vi "Drums Only.vi"() -> ()   [LabVIEW 2009]
uses:
  <vilib>/vision/Image Controls.llb/IMAQ Image.ctl
  <vilib>/Instr/_visa.llb/VISA Configure Serial Port (Instr).vi
  <vilib>/Analysis/3filter.llb/Filter Passband Type.ctl
  <vilib>/Analysis/3filter.llb/Butterworth Filter (DBL).vi
  <vilib>/vision/NI_Vision_Development_Module.lvlib
  <vilib>/Analysis/NI_AALBase.lvlib
panel:
  in  "Orange Guitar":T1={"Global Rectangle"=[220, 296, 225, 371], "Contours"=[{"ID"=enum."External", "Type"=2, "Coordinates"=[224, 370, 220, 296]}]} {"Contours"."Type" items=["No Selection", "Point", "Line", "Rectangle", "Oval", "Polygon", "Freehand Region", "Annulus", "Unused2", "Unused3", "Broken Line", "Freehand Line", "Rotated Rectangle"]}
  out "Orange Guitar":dbl[](graph)
  out "Orange Guitar LED":bool
  in  "sampling 8":dbl=1.0 format="%0.2f"
  in  "high 9":dbl=60.0 format="%0.2f"
  in  "low  8":dbl=0.12500000000000006 format="%0.4f"
  out "Orange Guitar":T1={"Global Rectangle"=[300, 297, 320, 380], "Contours"=[{"ID"=enum."External", "Type"=2, "Coordinates"=[300, 379, 319, 297]}]} {"Contours"."Type" items=["No Selection", "Point", "Line", "Rectangle", "Oval", "Polygon", "Freehand Region", "Annulus", "Unused2", "Unused3", "Broken Line", "Freehand Line", "Rotated Rectangle"]}
  in  "Green Guitar":T1={"Global Rectangle"=[100, 292, 131, 371], "Contours"=[{"ID"=enum."External", "Type"=2, "Coordinates"=[100, 370, 130, 292]}]} {"Contours"."Type" items=["No Selection", "Point", "Line", "Rectangle", "Oval", "Polygon", "Freehand Region", "Annulus", "Unused2", "Unused3", "Broken Line", "Freehand Line", "Rotated Rectangle"]}
  in  "Blue Guitar":T1={"Global Rectangle"=[193, 293, 199, 374], "Contours"=[{"ID"=enum."External", "Type"=2, "Coordinates"=[193, 373, 198, 293]}]} {"Contours"."Type" items=["No Selection", "Point", "Line", "Rectangle", "Oval", "Polygon", "Freehand Region", "Annulus", "Unused2", "Unused3", "Broken Line", "Freehand Line", "Rotated Rectangle"]}
  in  "Red Guitar":T1={"Global Rectangle"=[129, 294, 154, 376], "Contours"=[{"ID"=enum."External", "Type"=2, "Coordinates"=[129, 375, 153, 294]}]} {"Contours"."Type" items=["No Selection", "Point", "Line", "Rectangle", "Oval", "Polygon", "Freehand Region", "Annulus", "Unused2", "Unused3", "Broken Line", "Freehand Line", "Rotated Rectangle"]}
  in  "Yellow Guitar":T1={"Global Rectangle"=[160, 295, 175, 378], "Contours"=[{"ID"=enum."External", "Type"=2, "Coordinates"=[160, 377, 174, 295]}]} {"Contours"."Type" items=["No Selection", "Point", "Line", "Rectangle", "Oval", "Polygon", "Freehand Region", "Annulus", "Unused2", "Unused3", "Broken Line", "Freehand Line", "Rotated Rectangle"]}
  in  "sampling  8":dbl=1.0 format="%0.2f"
  in  "high 8":dbl=60.0 format="%0.2f"
  out "Blue Guitar":dbl[](graph)
  in  "low 2":dbl=0.12500000000000006 format="%0.4f"
  out "Yellow Guitar":dbl[](graph)
  out "Yellow Guitar LED":bool
  in  "sampling 7":dbl=1.0 format="%0.2f"
  in  "high 7":dbl=60.0 format="%0.2f"
  in  "low  7":dbl=0.12500000000000006 format="%0.4f"
  out "Yellow Guitar":T1={"Global Rectangle"=[243, 262, 261, 384], "Contours"=[{"ID"=enum."External", "Type"=2, "Coordinates"=[260, 383, 243, 262]}]} {"Contours"."Type" items=["No Selection", "Point", "Line", "Rectangle", "Oval", "Polygon", "Freehand Region", "Annulus", "Unused2", "Unused3", "Broken Line", "Freehand Line", "Rotated Rectangle"]}
  out "Blue Guitar":T1={"Global Rectangle"=[168, 264, 180, 378], "Contours"=[{"ID"=enum."External", "Type"=2, "Coordinates"=[168, 377, 179, 264]}]} {"Contours"."Type" items=["No Selection", "Point", "Line", "Rectangle", "Oval", "Polygon", "Freehand Region", "Annulus", "Unused2", "Unused3", "Broken Line", "Freehand Line", "Rotated Rectangle"]}
  out "Green Guitar":dbl[](graph)
  out "Green Guitar LED":bool
  in  "sampling 6":dbl=1.0 format="%0.2f"
  in  "high 6":dbl=60.0 format="%0.2f"
  in  "low  6":dbl=0.12500000000000006 format="%0.4f"
  out "Green Guitar":T1={"Global Rectangle"=[406, 309, 423, 383], "Contours"=[{"ID"=enum."External", "Type"=2, "Coordinates"=[422, 382, 406, 309]}]} {"Contours"."Type" items=["No Selection", "Point", "Line", "Rectangle", "Oval", "Polygon", "Freehand Region", "Annulus", "Unused2", "Unused3", "Broken Line", "Freehand Line", "Rotated Rectangle"]}
  out "Red Guitar":dbl[](graph)
  out "Red Guitar LED":bool
  in  "sampling 5":dbl=1.0 format="%0.2f"
  in  "high 5":dbl=60.0 format="%0.2f"
  in  "low  5":dbl=0.12500000000000006 format="%0.4f"
  out "Red Guitar":T1={"Global Rectangle"=[300, 297, 320, 380], "Contours"=[{"ID"=enum."External", "Type"=2, "Coordinates"=[300, 379, 319, 297]}]} {"Contours"."Type" items=["No Selection", "Point", "Line", "Rectangle", "Oval", "Polygon", "Freehand Region", "Annulus", "Unused2", "Unused3", "Broken Line", "Freehand Line", "Rotated Rectangle"]}
  out "Blue Guitar LED":bool
  in  "Mask":T1 {"Contours"."Type" items=["No Selection", "Point", "Line", "Rectangle", "Oval", "Polygon", "Freehand Region", "Annulus", "Unused2", "Unused3", "Broken Line", "Freehand Line", "Rotated Rectangle"]}
  out "Image 2":T2(plugin-control)
  out "Red Line":T1={"Global Rectangle"=[300, 297, 320, 380], "Contours"=[{"ID"=enum."External", "Type"=2, "Coordinates"=[300, 379, 319, 297]}]} {"Contours"."Type" items=["No Selection", "Point", "Line", "Rectangle", "Oval", "Polygon", "Freehand Region", "Annulus", "Unused2", "Unused3", "Broken Line", "Freehand Line", "Rotated Rectangle"]}
  in  "Red Line":T1={"Global Rectangle"=[300, 297, 320, 380], "Contours"=[{"ID"=enum."External", "Type"=2, "Coordinates"=[300, 379, 319, 297]}]} {"Contours"."Type" items=["No Selection", "Point", "Line", "Rectangle", "Oval", "Polygon", "Freehand Region", "Annulus", "Unused2", "Unused3", "Broken Line", "Freehand Line", "Rotated Rectangle"]}
  out "Waveform Red":dbl[](graph)
  out "LED Red":bool
  in  "sampling 4":dbl=1.0 format="%0.2f"
  in  "high 4":dbl=60.0 format="%0.2f"
  in  "low  4":dbl=0.12500000000000006 format="%0.4f"
  out "Green Line":T1={"Global Rectangle"=[406, 309, 423, 383], "Contours"=[{"ID"=enum."External", "Type"=2, "Coordinates"=[422, 382, 406, 309]}]} {"Contours"."Type" items=["No Selection", "Point", "Line", "Rectangle", "Oval", "Polygon", "Freehand Region", "Annulus", "Unused2", "Unused3", "Broken Line", "Freehand Line", "Rotated Rectangle"]}
  in  "Blue Line":T1={"Global Rectangle"=[374, 278, 383, 377], "Contours"=[{"ID"=enum."External", "Type"=2, "Coordinates"=[382, 376, 374, 278]}]} {"Contours"."Type" items=["No Selection", "Point", "Line", "Rectangle", "Oval", "Polygon", "Freehand Region", "Annulus", "Unused2", "Unused3", "Broken Line", "Freehand Line", "Rotated Rectangle"]}
  in  "Green Line":T1={"Global Rectangle"=[406, 309, 423, 383], "Contours"=[{"ID"=enum."External", "Type"=2, "Coordinates"=[422, 382, 406, 309]}]} {"Contours"."Type" items=["No Selection", "Point", "Line", "Rectangle", "Oval", "Polygon", "Freehand Region", "Annulus", "Unused2", "Unused3", "Broken Line", "Freehand Line", "Rotated Rectangle"]}
  in  "low  3":dbl=0.12500000000000006 format="%0.4f"
  out "Waveform Green":dbl[](graph)
  out "LED Green":bool
  in  "sampling 3":dbl=1.0 format="%0.2f"
  in  "high 3":dbl=60.0 format="%0.2f"
  in  "Yellow Line":T1={"Global Rectangle"=[342, 292, 349, 377], "Contours"=[{"ID"=enum."External", "Type"=2, "Coordinates"=[342, 376, 348, 292]}]} {"Contours"."Type" items=["No Selection", "Point", "Line", "Rectangle", "Oval", "Polygon", "Freehand Region", "Annulus", "Unused2", "Unused3", "Broken Line", "Freehand Line", "Rotated Rectangle"]}
  out "Blue Line":T1={"Global Rectangle"=[168, 264, 180, 378], "Contours"=[{"ID"=enum."External", "Type"=2, "Coordinates"=[168, 377, 179, 264]}]} {"Contours"."Type" items=["No Selection", "Point", "Line", "Rectangle", "Oval", "Polygon", "Freehand Region", "Annulus", "Unused2", "Unused3", "Broken Line", "Freehand Line", "Rotated Rectangle"]}
  out "cluster":T3
  in  "baud rate (9600)":u32=9600
  in  "VISA resource name":refnum<visa-resource-name>
  out "number":u8
  out "decimal integer string":string
  out "Image Dst Out":T2
  out "Yellow Line":T1={"Global Rectangle"=[243, 262, 261, 384], "Contours"=[{"ID"=enum."External", "Type"=2, "Coordinates"=[260, 383, 243, 262]}]} {"Contours"."Type" items=["No Selection", "Point", "Line", "Rectangle", "Oval", "Polygon", "Freehand Region", "Annulus", "Unused2", "Unused3", "Broken Line", "Freehand Line", "Rotated Rectangle"]}
  in  "low  2":dbl=0.12500000000000006 format="%0.4f"
  in  "high 2":dbl=60.0 format="%0.2f"
  in  "sampling 2":dbl=1.0 format="%0.2f"
  out "LED Yellow":bool
  out "Waveform Yellow":dbl[](graph)
  in  "playtime":dbl=30.0
  out "Frame Number":i32
  in  "Frame Start":i32=2400
  out "Blue Drum":bool
  in  "low":dbl=0.12500000000000006 format="%0.4f"
  out "Blue Drum":dbl[](graph)
  in  "high":dbl=60.0 format="%0.2f"
  in  "sampling":dbl=1.0 format="%0.2f"
  in  "stop":bool
  in  "AVI Path":path
  # "BLUE"
  # "YELLOW"
  # "GREEN"
  # "RED"
  # "Drums"
  # "Guitar"
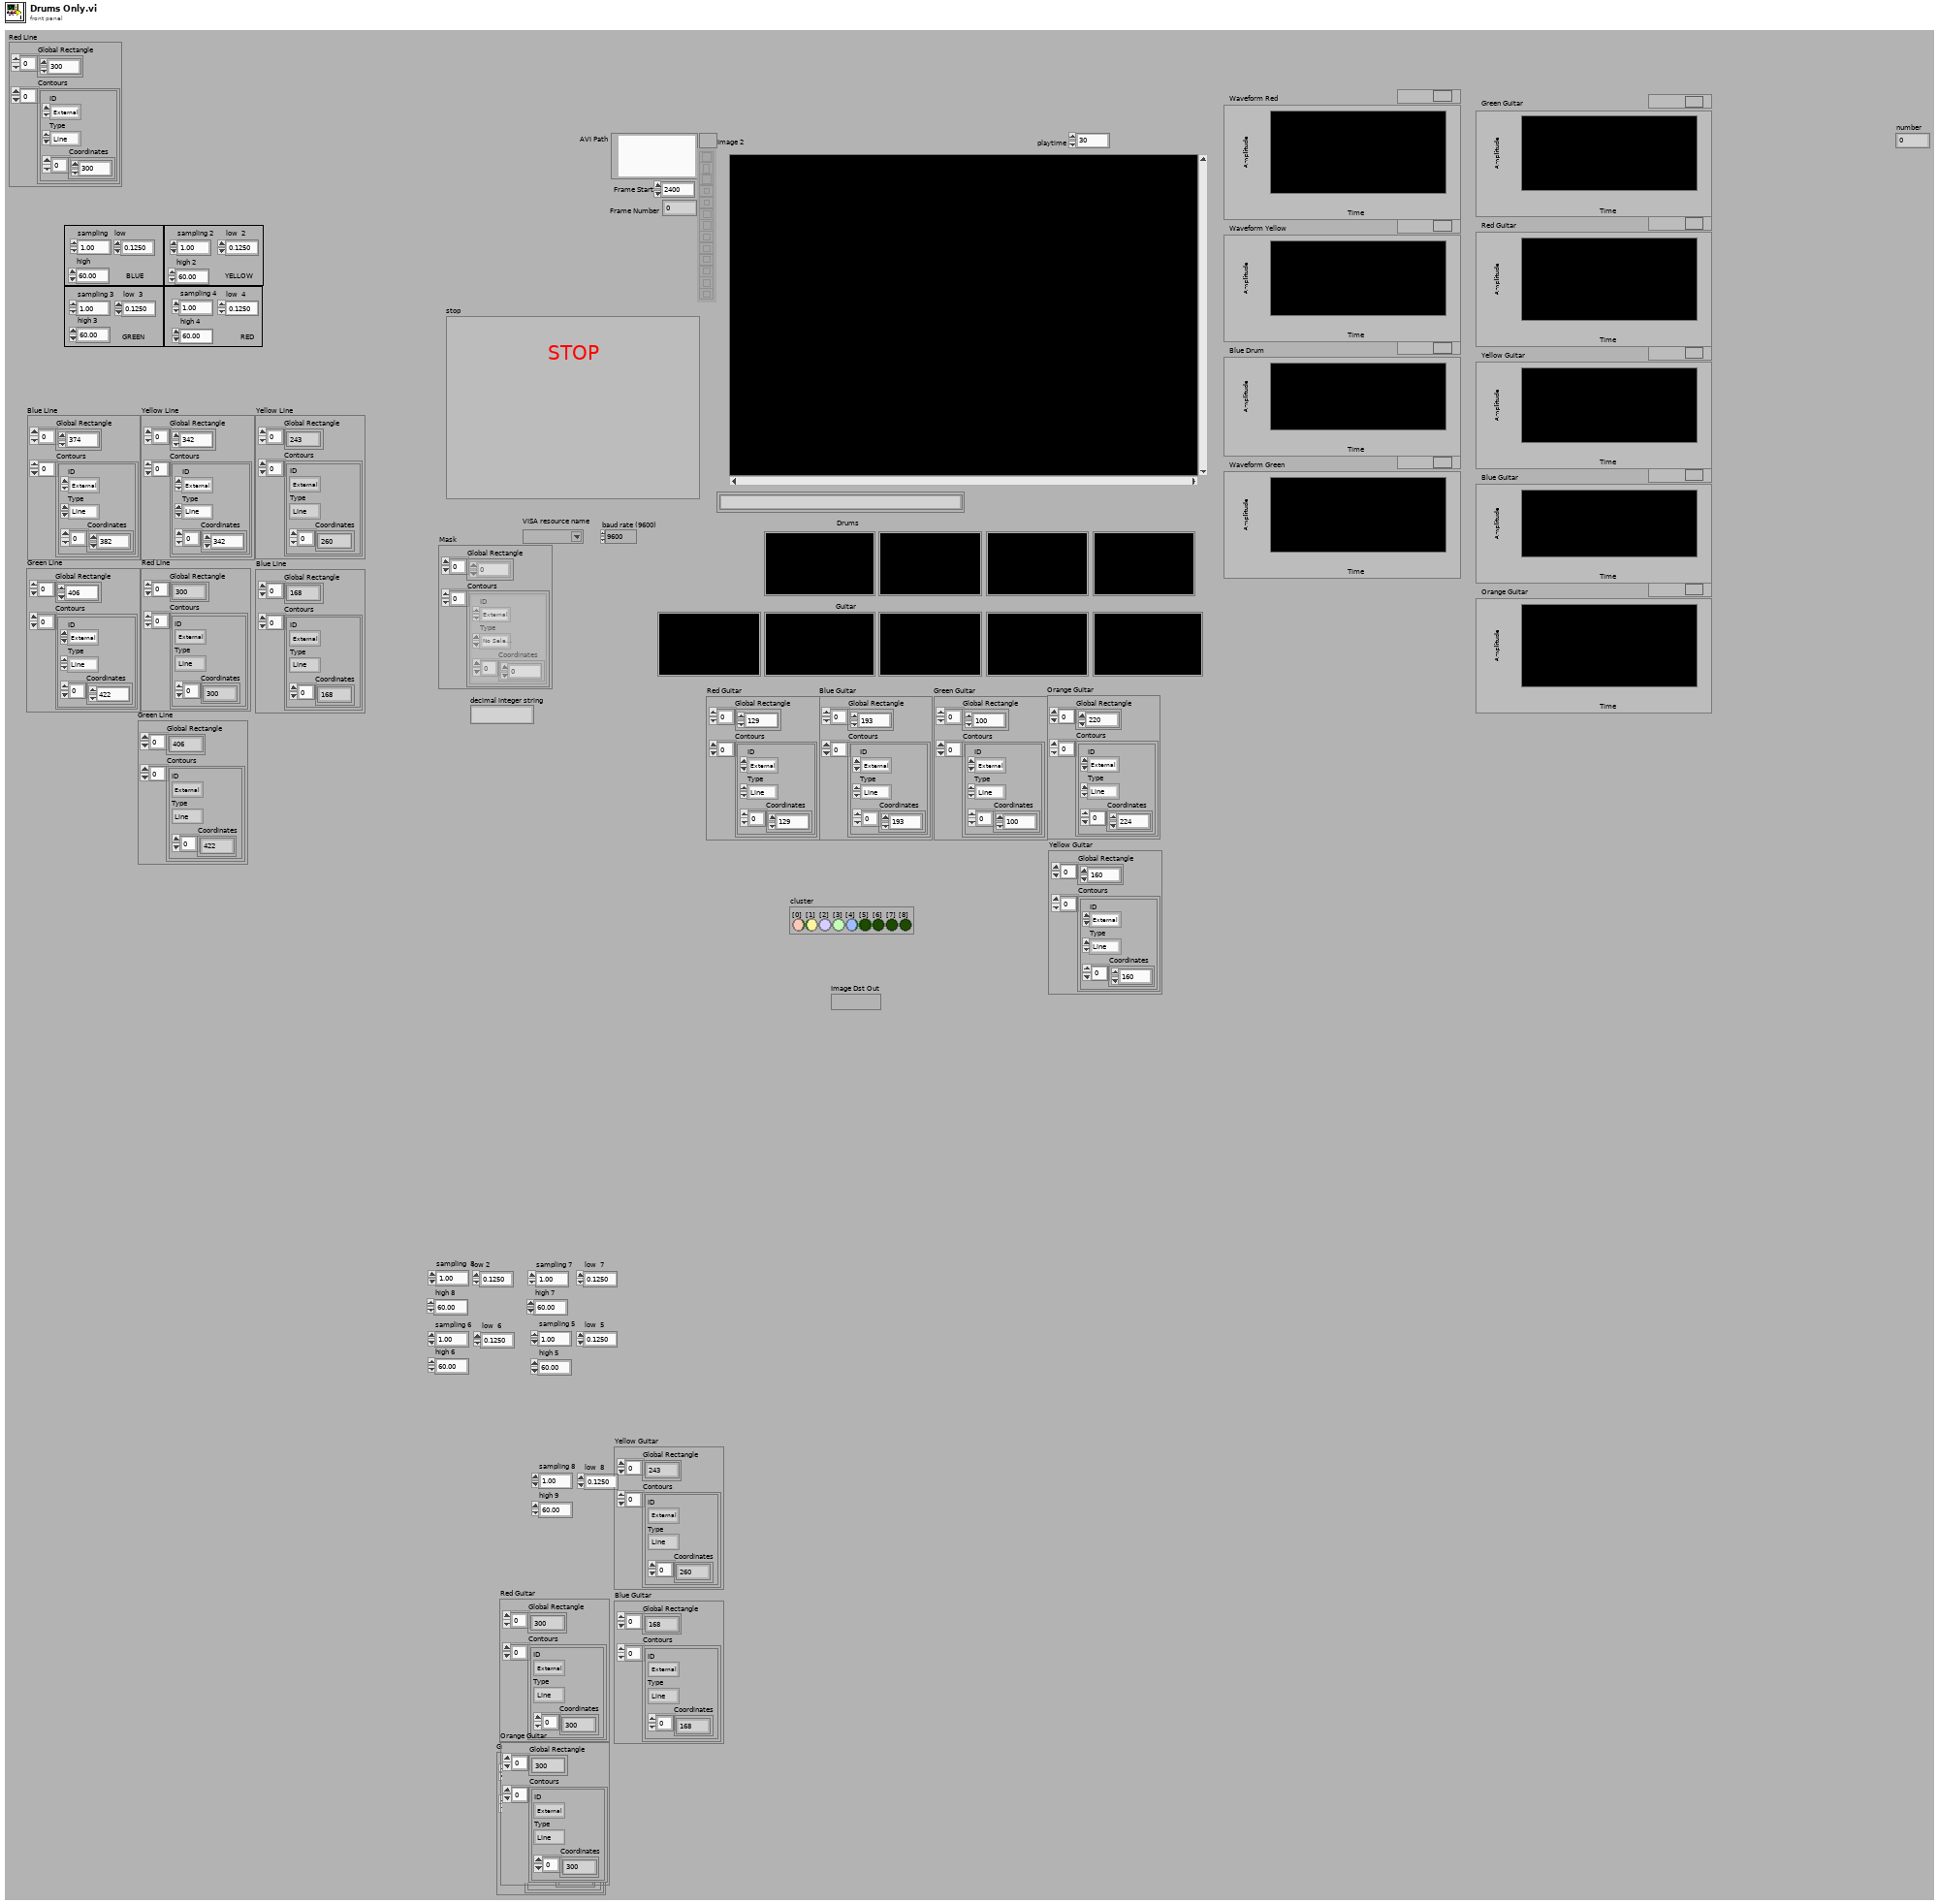
[diagram p1: front panel]
types:
  T1 = cluster{"Global Rectangle":i32[], "Contours":cluster{"ID":enum32{"External", "Internal"}, "Type":u32, "Coordinates":i32[]}[]}
  T2 = typedef "IMAQ Image.ctl" = refnum<image>
  T3 = cluster{"[0]":bool, "[1]":bool, "[2]":bool, "[3]":bool, "[4]":bool, "[5]":bool, "[6]":bool, "[7]":bool, "[8]":bool}
  T4 = typedef "NI_AALBase.lvlib/Filter Passband Type.ctl" = enum32{"Lowpass", "Highpass", "Bandpass", "Bandstop"}
  T5 = cluster{"Left":i32, "Top":i32, "Right":i32, "Bottom":i32}
  T6 = typedef "Image Type" = u32
  T7 = typedef "AviRefnum.ctl" = refnum<k1>
  T8 = cluster{"ID":enum32{"External", "Internal"}, "Type":u32, "Coordinates":i32[]}[]
  T9 = cluster{"ID":enum32{"External", "Internal"}, "Type":u32, "Coordinates":i32[]}
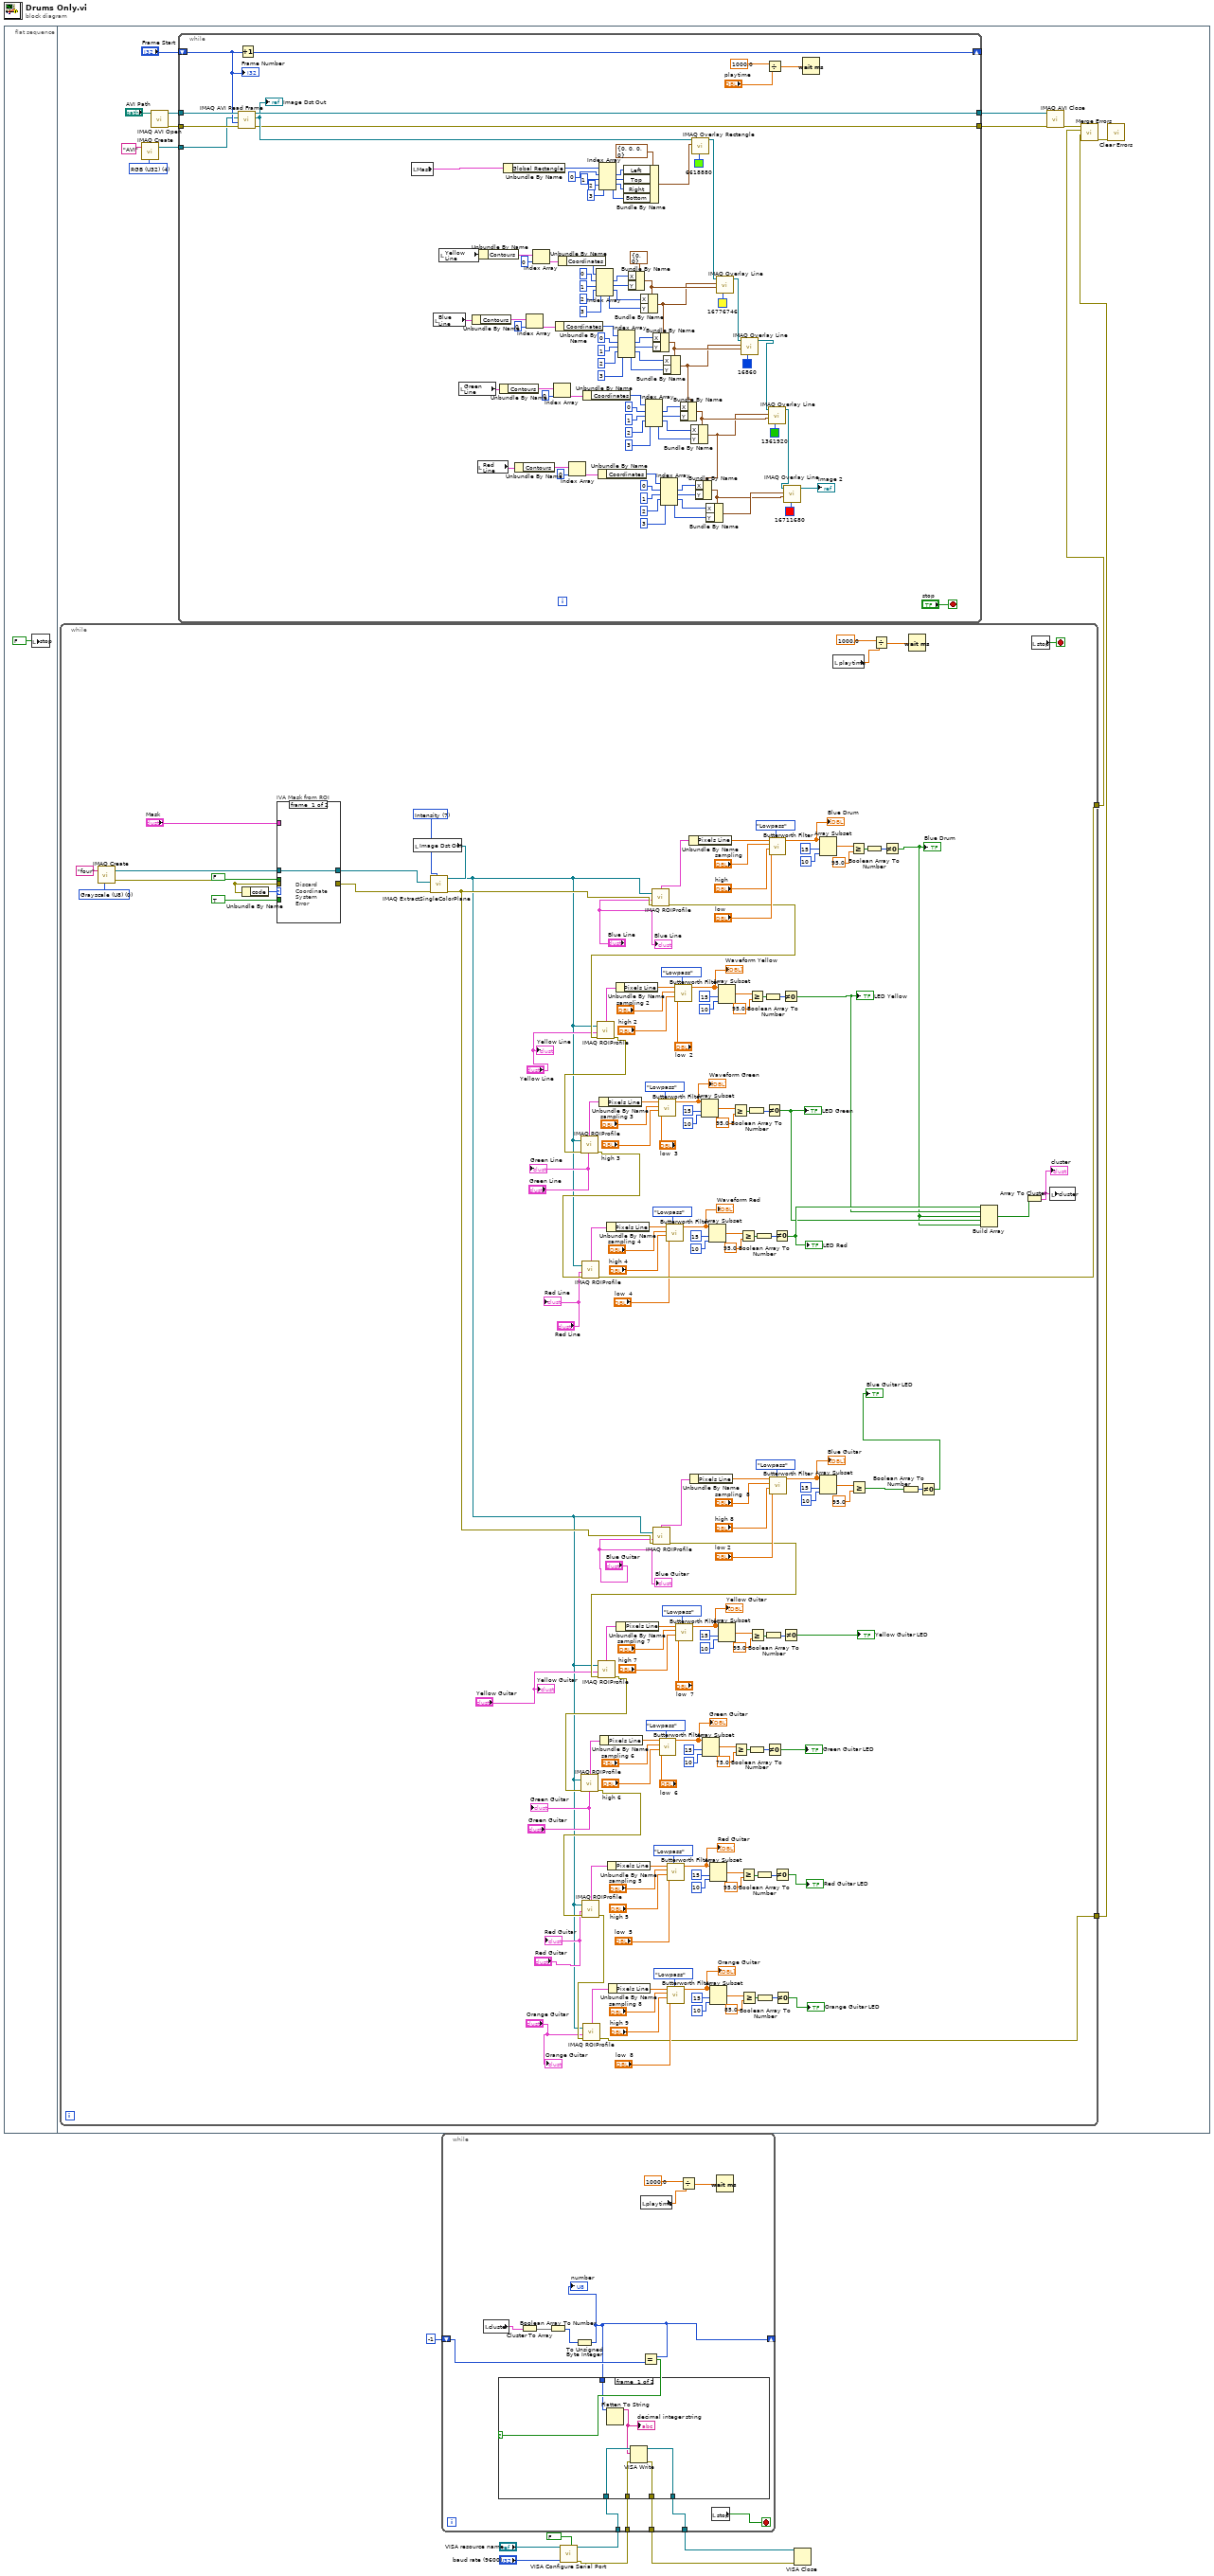
[diagram p0: block diagram]
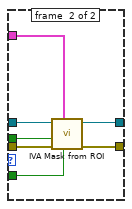
[diagram p3: hidden frame]
diagram:
  n1 = flat-sequence {
    frame #0 {
      n2 = local write "stop"(FALSE ("stop")) -> ()
    }
    frame #1 {
      w14 = T6 4 items=["Grayscale (U8)", "Grayscale (I16)", "Grayscale (SGL)", "Complex (CSG)", "RGB (U32)", "HSL (U32)", "RGB (U64)", "Grayscale (U16)"] ("Image Type")
      n3 = while {
        tunnel: [w170] -> w11
        tunnel: [w35] -> w10
        stop <- w185 stop-if-true
        w180 = T6 0 items=["Grayscale (U8)", "Grayscale (I16)", "Grayscale (SGL)", "Complex (CSG)", "RGB (U32)", "HSL (U32)", "RGB (U64)", "Grayscale (U16)"] ("Image Type")
        w186 = 7 items=["Red", "Green", "Blue", "Hue", "Saturation", "Luminance", "Value", "Intensity"] ("Color Plane")
        n4 = call "IMAQ Create"("Image Name"="four", "Image Type"=w180) -> ("New Image"=w173:T2, "error out"=w174:errorcluster)  [unwired: 3 in]
        n5 = Unbundle By Name(w174) -> ("code"=w178:i32)
        n6 = case "IVA Mask from ROI" shown="Default" w178 {
          tunnel: "Mask" -> [_ w194]
          tunnel: TRUE ("Shrink") -> [_ w193]
          tunnel: w173 -> [w187 w192]
          tunnel: w174 -> [_ w191]
          tunnel: [_ w190] -> w175
          tunnel: [w187 w189] -> w171
          tunnel: FALSE ("Out / In") -> [_ w188]
          frame #0 {
            # "Discard\nCoordinate\nSystem\nError"
          }
          frame #1 {
            n7 = call <vilib>:"IVA Mask from ROI.vi"("Shrink"=w193, "ROI Descriptor"=w194, "error in (no error)"=w191, "Out / In"=w188, "Image Src"=w192) -> ("error out"=w190:errorcluster, "Image Out"=w189:T2)  [unwired: 5 out]
          }
        }
        n8 = local read "Image Dst Out"() -> (w181:T2)
        n9 = call "IMAQ ExtractSingleColorPlane"("Color Plane"=w186, "error in (no error)"=w175, "Image Dst"=w171, "Image Src"=w181) -> ("error out"=w169:errorcluster, "Image Dst Out"=w34:T2)  [unwired: 6 out]
        n10 = call "IMAQ ROIProfile"("error in (no error)"=w169, "ROI Descriptor"="Blue Line", "Image"=w34) -> ("error out"=w144:errorcluster, "ROI Graph"=w143:cluster{"x0":sgl, "dx":sgl, "Pixels Line":sgl[]})  [unwired: 4 out]
        n11 = call "IMAQ ROIProfile"("error in (no error)"=w144, "ROI Descriptor"="Yellow Line", "Image"=w34) -> ("error out"=w111:errorcluster, "ROI Graph"=w147:cluster{"x0":sgl, "dx":sgl, "Pixels Line":sgl[]})  [unwired: 4 out]
        n12 = call "IMAQ ROIProfile"("error in (no error)"=w111, "ROI Descriptor"="Green Line", "Image"=w34) -> ("error out"=w114:errorcluster, "ROI Graph"=w141:cluster{"x0":sgl, "dx":sgl, "Pixels Line":sgl[]})  [unwired: 4 out]
        n13 = call "IMAQ ROIProfile"("error in (no error)"=w114, "ROI Descriptor"="Red Line", "Image"=w34) -> ("error out"=w170:errorcluster, "ROI Graph"=w116:cluster{"x0":sgl, "dx":sgl, "Pixels Line":sgl[]})  [unwired: 4 out]
        n14 = Unbundle By Name(w141) -> ("Pixels Line"=w138:sgl[])
        n15 = Unbundle By Name(w116) -> ("Pixels Line"=w119:sgl[])
        n16 = Unbundle By Name(w147) -> ("Pixels Line"=w150:sgl[])
        n17 = call "IMAQ ROIProfile"("error in (no error)"=w169, "ROI Descriptor"="Blue Guitar", "Image"=w34) -> ("error out"=w84:errorcluster, "ROI Graph"=w83:cluster{"x0":sgl, "dx":sgl, "Pixels Line":sgl[]})  [unwired: 4 out]
        n18 = call "IMAQ ROIProfile"("error in (no error)"=w84, "ROI Descriptor"="Yellow Guitar", "Image"=w34) -> ("error out"=w54:errorcluster, "ROI Graph"=w87:cluster{"x0":sgl, "dx":sgl, "Pixels Line":sgl[]})  [unwired: 4 out]
        n19 = call "IMAQ ROIProfile"("error in (no error)"=w54, "ROI Descriptor"="Green Guitar", "Image"=w34) -> ("error out"=w55:errorcluster, "ROI Graph"=w81:cluster{"x0":sgl, "dx":sgl, "Pixels Line":sgl[]})  [unwired: 4 out]
        n20 = call "IMAQ ROIProfile"("error in (no error)"=w55, "ROI Descriptor"="Red Guitar", "Image"=w34) -> ("error out"=w36:errorcluster, "ROI Graph"=w57:cluster{"x0":sgl, "dx":sgl, "Pixels Line":sgl[]})  [unwired: 4 out]
        n21 = call "IMAQ ROIProfile"("error in (no error)"=w36, "ROI Descriptor"="Orange Guitar", "Image"=w34) -> ("error out"=w35:errorcluster, "ROI Graph"=w48:cluster{"x0":sgl, "dx":sgl, "Pixels Line":sgl[]})  [unwired: 4 out]
        n22 = Unbundle By Name(w81) -> ("Pixels Line"=w78:sgl[])
        n23 = Unbundle By Name(w57) -> ("Pixels Line"=w60:sgl[])
        n24 = Unbundle By Name(w48) -> ("Pixels Line"=w45:sgl[])
        n25 = Unbundle By Name(w87) -> ("Pixels Line"=w90:sgl[])
        n26 = call-poly <vilib>:"Butterworth Filter.vi"("filter type"=Filter_Passband_Type."Lowpass", "low cutoff freq: fl"="low  3", "high cutoff freq: fh"="high 3", "sampling freq: fs"="sampling 3", "X"=w138) -> ("Filtered X"=w142:dbl[])  [unwired: 3 in, 1 out]
        "Waveform Green" <- w142
        n27 = call-poly <vilib>:"Butterworth Filter.vi"("filter type"=Filter_Passband_Type."Lowpass", "low cutoff freq: fl"="low  6", "high cutoff freq: fh"="high 6", "sampling freq: fs"="sampling 6", "X"=w78) -> ("Filtered X"=w82:dbl[])  [unwired: 3 in, 1 out]
        "Green Guitar" <- w82
        n28 = call-poly <vilib>:"Butterworth Filter.vi"("filter type"=Filter_Passband_Type."Lowpass", "low cutoff freq: fl"="low  4", "high cutoff freq: fh"="high 4", "sampling freq: fs"="sampling 4", "X"=w119) -> ("Filtered X"=w115:dbl[])  [unwired: 3 in, 1 out]
        "Waveform Red" <- w115
        n29 = call-poly <vilib>:"Butterworth Filter.vi"("filter type"=Filter_Passband_Type."Lowpass", "low cutoff freq: fl"="low  5", "high cutoff freq: fh"="high 5", "sampling freq: fs"="sampling 5", "X"=w60) -> ("Filtered X"=w56:dbl[])  [unwired: 3 in, 1 out]
        "Red Guitar" <- w56
        n30 = call-poly <vilib>:"Butterworth Filter.vi"("filter type"=Filter_Passband_Type."Lowpass", "low cutoff freq: fl"="low  8", "high cutoff freq: fh"="high 9", "sampling freq: fs"="sampling 8", "X"=w45) -> ("Filtered X"=w49:dbl[])  [unwired: 3 in, 1 out]
        "Orange Guitar" <- w49
        n31 = call-poly <vilib>:"Butterworth Filter.vi"("filter type"=Filter_Passband_Type."Lowpass", "low cutoff freq: fl"="low  2", "high cutoff freq: fh"="high 2", "sampling freq: fs"="sampling 2", "X"=w150) -> ("Filtered X"=w146:dbl[])  [unwired: 3 in, 1 out]
        "Waveform Yellow" <- w146
        n32 = call-poly <vilib>:"Butterworth Filter.vi"("filter type"=Filter_Passband_Type."Lowpass", "low cutoff freq: fl"="low  7", "high cutoff freq: fh"="high 7", "sampling freq: fs"="sampling 7", "X"=w90) -> ("Filtered X"=w86:dbl[])  [unwired: 3 in, 1 out]
        "Yellow Guitar" <- w86
        n33 = Unbundle By Name(w143) -> ("Pixels Line"=w167:sgl[])
        n34 = Unbundle By Name(w83) -> ("Pixels Line"=w106:sgl[])
        n35 = Array Subset(array=w142, index=15, length=10) -> (w133:dbl[])
        n36 = Array Subset(array=w82, index=15, length=10) -> (w73:dbl[])
        n37 = Array Subset(array=w115, index=15, length=10) -> (w124:dbl[])
        n38 = Array Subset(array=w56, index=15, length=10) -> (w65:dbl[])
        n39 = Array Subset(array=w49, index=15, length=10) -> (w40:dbl[])
        n40 = Array Subset(array=w146, index=15, length=10) -> (w155:dbl[])
        n41 = Array Subset(array=w86, index=15, length=10) -> (w95:dbl[])
        n42 = Greater Or Equal?(x=w133, y=95.0) -> (x >= y?=w135:bool[])
        n43 = Greater Or Equal?(x=w73, y=75.0) -> (x >= y?=w75:bool[])
        n44 = Greater Or Equal?(x=w124, y=95.0) -> (x >= y?=w122:bool[])
        n45 = Greater Or Equal?(x=w65, y=95.0) -> (x >= y?=w63:bool[])
        n46 = Greater Or Equal?(x=w40, y=85.0) -> (x >= y?=w42:bool[])
        n47 = Boolean Array To Number(Boolean array=w135) -> (number=w136:u32)
        n48 = Greater Or Equal?(x=w155, y=95.0) -> (x >= y?=w153:bool[])
        n49 = Boolean Array To Number(Boolean array=w75) -> (number=w76:u32)
        n50 = Greater Or Equal?(x=w95, y=95.0) -> (x >= y?=w93:bool[])
        n51 = Boolean Array To Number(Boolean array=w122) -> (number=w121:u32)
        n52 = Boolean Array To Number(Boolean array=w63) -> (number=w62:u32)
        n53 = Boolean Array To Number(Boolean array=w42) -> (number=w43:u32)
        n54 = Boolean Array To Number(Boolean array=w153) -> (number=w152:u32)
        n55 = Boolean Array To Number(Boolean array=w93) -> (number=w92:u32)
        n56 = Not Equal To 0?(x=w136) -> (x != 0?=w24:bool)
        "LED Green" <- w24
        n57 = Not Equal To 0?(x=w76) -> (x != 0?=→"Green Guitar LED":bool)
        n58 = call-poly <vilib>:"Butterworth Filter.vi"("filter type"=Filter_Passband_Type."Lowpass", "low cutoff freq: fl"="low", "high cutoff freq: fh"="high", "sampling freq: fs"="sampling", "X"=w167) -> ("Filtered X"=w129:dbl[])  [unwired: 3 in, 1 out]
        "Blue Drum" <- w129
        n59 = call-poly <vilib>:"Butterworth Filter.vi"("filter type"=Filter_Passband_Type."Lowpass", "low cutoff freq: fl"="low 2", "high cutoff freq: fh"="high 8", "sampling freq: fs"="sampling  8", "X"=w106) -> ("Filtered X"=w69:dbl[])  [unwired: 3 in, 1 out]
        "Blue Guitar" <- w69
        n60 = Not Equal To 0?(x=w121) -> (x != 0?=w26:bool)
        "LED Red" <- w26
        n61 = Not Equal To 0?(x=w62) -> (x != 0?=→"Red Guitar LED":bool)
        n62 = Not Equal To 0?(x=w43) -> (x != 0?=→"Orange Guitar LED":bool)
        n63 = Not Equal To 0?(x=w152) -> (x != 0?=w25:bool)
        "LED Yellow" <- w25
        n64 = Not Equal To 0?(x=w92) -> (x != 0?=→"Yellow Guitar LED":bool)
        n65 = Array Subset(array=w129, index=15, length=10) -> (w161:dbl[])
        n66 = Array Subset(array=w69, index=15, length=10) -> (w100:dbl[])
        n67 = local read "playtime"() -> (w182:dbl)
        n68 = Greater Or Equal?(x=w161, y=95.0) -> (x >= y?=w159:bool[])
        n69 = Greater Or Equal?(x=w100, y=95.0) -> (x >= y?=w27:bool[])
        n70 = Boolean Array To Number(Boolean array=w159) -> (number=w158:u32)
        n71 = Divide(x=1000.0, y=w182) -> (x/y=w184:dbl)
        n72 = Not Equal To 0?(x=w158) -> (x != 0?=w23:bool)
        "Blue Drum" <- w23
        n73 = Boolean Array To Number(Boolean array=w27) -> (number=w98:u32)
        n74 = Wait (ms)(milliseconds to wait=w184) -> ()  [unwired: 1 out]
        n75 = Not Equal To 0?(x=w98) -> (x != 0?=→"Blue Guitar LED":bool)
        n76 = Build Array(w26, w25, w23, w24, w23) -> (w109:bool[])
        n77 = Array To Cluster(array=w109) -> (cluster=w110:T3)
        "cluster" <- w110
        n78 = local read "stop"() -> (w185:bool)
        n79 = local write "cluster"(w110) -> ()
        "Yellow Line" <- "Yellow Line"
        "Blue Line" <- "Blue Line"
        "Green Line" <- "Green Line"
        "Red Line" <- "Red Line"
        "Yellow Guitar" <- "Yellow Guitar"
        "Blue Guitar" <- "Blue Guitar"
        "Green Guitar" <- "Green Guitar"
        "Red Guitar" <- "Red Guitar"
        "Orange Guitar" <- "Orange Guitar"
      }
      n80 = call "IMAQ Create"("Image Name"="AVI", "Image Type"=w14) -> ("New Image"=w12:T2)  [unwired: 3 in, 1 out]
      n81 = call "IMAQ AVI Open"("AVI Path"="AVI Path") -> ("error out"=w19:errorcluster, "Avi Refnum"=w20:T7)  [unwired: 9 in]
      n82 = while {
        tunnel: w20 -> [w289]
        tunnel: w19 -> [w237]
        tunnel: [w288] -> w21
        shift-right: [w283] -> _
        shift-left: "Frame Start" -> [w282]
        tunnel: [w233] -> w15
        tunnel: w12 -> [w232]
        stop <- "stop" stop-if-true
        n83 = call "IMAQ AVI Read Frame"("error in (no error)"=w237, "Frame Number"=w282, "Image"=w232, "Avi Refnum"=w289) -> ("error out"=w233:errorcluster, "Image Out"=w234:T2, "Avi Refnum (duplicate)"=w288:T7)  [unwired: 4 in, 1 out]
        "Image Dst Out" <- w234
        n84 = Increment(x=w282) -> (x+1=w283:i32)
        n85 = local read "Mask"() -> (w195:T1)
        n86 = local read "Blue Line"() -> (w236:T1)
        n87 = local read "Yellow Line"() -> (w235:T1)
        n88 = local read "Green Line"() -> (w231:T1)
        n89 = Unbundle By Name(w236) -> ("Contours"=w249:T8)
        n90 = local read "Red Line"() -> (w198:T1)
        n91 = Unbundle By Name(w235) -> ("Contours"=w264:T8)
        n92 = Unbundle By Name(w231) -> ("Contours"=w221:T8)
        n93 = Unbundle By Name(w195) -> ("Global Rectangle"=w278:i32[])
        n94 = Unbundle By Name(w198) -> ("Contours"=w208:T8)
        n95 = Index Array(array=w249, index=0) -> (element=w248:T9)
        n96 = Index Array(array=w264, index=0) -> (element=w266:T9)
        n97 = Index Array(array=w221, index=0) -> (element=w222:T9)
        n98 = Unbundle By Name(w248) -> ("Coordinates"=w247:i32[])
        n99 = Unbundle By Name(w266) -> ("Coordinates"=w267:i32[])
        n100 = Index Array(array=w208, index=0) -> (element=w207:T9)
        n101 = Unbundle By Name(w222) -> ("Coordinates"=w223:i32[])
        n102 = Index Array(array=w267, index #1=0 ("index"), index #2=1 ("index"), index #3=2 ("index"), index #4=3 ("index")) -> (element #1=w259:i32, element #2=w260:i32, element #3=w261:i32, element #4=w262:i32)
        n103 = Unbundle By Name(w207) -> ("Coordinates"=w206:i32[])
        n104 = Index Array(array=w278, index #1=0 ("index"), index #2=1 ("index"), index #3=2 ("index"), index #4=3 ("index")) -> (element #1=w277:i32, element #2=w276:i32, element #3=w275:i32, element #4=w274:i32)
        n105 = Index Array(array=w247, index #1=0 ("index"), index #2=1 ("index"), index #3=2 ("index"), index #4=3 ("index")) -> (element #1=w246:i32, element #2=w252:i32, element #3=w251:i32, element #4=w250:i32)
        n106 = Bundle By Name(cluster=T5 {"Left"=0, "Top"=0, "Right"=0, "Bottom"=0} ("Rectangle"), "Left"=w277, "Top"=w276, "Right"=w275, "Bottom"=w274) -> (w280:T5)
        n107 = Bundle By Name(cluster=cluster{"X":i32, "Y":i32} {"X"=0, "Y"=0} ("End Point"), "X"=w259, "Y"=w260) -> (w268:cluster{"X":i32, "Y":i32})
        n108 = Bundle By Name(cluster=w268, "X"=w261, "Y"=w262) -> (w239:cluster{"X":i32, "Y":i32})
        n109 = Index Array(array=w223, index #1=0 ("index"), index #2=1 ("index"), index #3=2 ("index"), index #4=3 ("index")) -> (element #1=w224:i32, element #2=w218:i32, element #3=w219:i32, element #4=w220:i32)
        n110 = Bundle By Name(cluster=w239, "X"=w246, "Y"=w252) -> (w253:cluster{"X":i32, "Y":i32})
        n111 = Index Array(array=w206, index #1=0 ("index"), index #2=1 ("index"), index #3=2 ("index"), index #4=3 ("index")) -> (element #1=w205:i32, element #2=w211:i32, element #3=w210:i32, element #4=w209:i32)
        n112 = Bundle By Name(cluster=w253, "X"=w251, "Y"=w250) -> (w216:cluster{"X":i32, "Y":i32})
        n113 = Bundle By Name(cluster=w216, "X"=w224, "Y"=w218) -> (w215:cluster{"X":i32, "Y":i32})
        n114 = Bundle By Name(cluster=w215, "X"=w219, "Y"=w220) -> (w197:cluster{"X":i32, "Y":i32})
        n115 = call "IMAQ Overlay Rectangle"("Color"=u32 6618880, "Rectangle"=w280, "Image"=w234) -> ("Image Out"=w254:T2)  [unwired: 7 in, 1 out]
        n116 = Bundle By Name(cluster=w197, "X"=w205, "Y"=w211) -> (w213:cluster{"X":i32, "Y":i32})
        n117 = Bundle By Name(cluster=w213, "X"=w210, "Y"=w209) -> (w214:cluster{"X":i32, "Y":i32})
        n118 = call "IMAQ Overlay Line"("Color"=u32 16776746, "End Point"=w268, "Start Point"=w239, "Image"=w254) -> ("Image Out"=w244:T2)  [unwired: 6 in, 1 out]
        n119 = call "IMAQ Overlay Line"("Color"=u32 16860, "End Point"=w253, "Start Point"=w216, "Image"=w244) -> ("Image Out"=w217:T2)  [unwired: 6 in, 1 out]
        n120 = Divide(x=1000.0, y="playtime") -> (x/y=w286:dbl)
        n121 = call "IMAQ Overlay Line"("Color"=u32 1361920, "End Point"=w215, "Start Point"=w197, "Image"=w217) -> ("Image Out"=w196:T2)  [unwired: 6 in, 1 out]
        n122 = call "IMAQ Overlay Line"("Color"=u32 16711680, "End Point"=w213, "Start Point"=w214, "Image"=w196) -> ("Image Out"=→"Image 2":T2)  [unwired: 6 in, 1 out]
        n123 = Wait (ms)(milliseconds to wait=w286) -> ()  [unwired: 1 out]
        "Frame Number" <- w282
      }
      n124 = call "IMAQ AVI Close"("error in (no error)"=w15, "Avi Refnum"=w21) -> ("error out"=w17:errorcluster)  [unwired: 9 in]
      n125 = call <vilib>:"Merge Errors.vi"("error in 3 (no error)"=w10, "error in 2 (no error)"=w11, "error in 1 (no error)"=w17) -> ("error out"=w16:errorcluster)  [unwired: 4 in]
      n126 = call <vilib>:"Clear Errors.vi"("error in (no error)"=w16) -> ()  [unwired: 6 in, 1 out]
    }
  }
  n127 = call-poly "VISA Configure Serial Port"("VISA resource name"="VISA resource name", "Enable Termination\nChar (T)"=FALSE ("Enable Termination\nChar (T)"), "baud rate (9600)"="baud rate (9600)") -> ("VISA resource name out"=w7:refnum<visa-resource-name>, "error out"=w2:errorcluster)  [unwired: 11 in]
  n128 = while {
    shift-right: [w290] -> _
    shift-left: -1 -> [w303]
    tunnel: w7 -> [w301]
    tunnel: [w300] -> w6
    tunnel: w2 -> [w299]
    tunnel: [w298] -> w1
    stop <- w295 stop-if-true
    n129 = local read "cluster"() -> (w296:T3)
    n130 = Cluster To Array(cluster=w296) -> (array=w297:bool[])
    n131 = Boolean Array To Number(Boolean array=w297) -> (number=w291:u32)
    n132 = To Unsigned Byte Integer(number=w291) -> (unsigned 8bit integer=w290:u8)
    "number" <- w290
    n133 = local read "playtime"() -> (w294:dbl)
    n134 = Equal?(x=w290, y=w303) -> (x = y?=w302:bool)
    n135 = case shown="False" w302 {
      tunnel: w301 -> [w309 w311]
      tunnel: [w308 w311] -> w300
      tunnel: w290 -> [w305 _]
      tunnel: w299 -> [w307 w310]
      tunnel: [w306 w310] -> w298
      frame #0 {
        n136 = Flatten To String(anything=w305) -> (data string=w304:string)  [unwired: 3 in, 2 out]
        "decimal integer string" <- w304
        n137 = VISA Write(VISA resource name=w309, write buffer=w304, error in (no error)=w307) -> (VISA resource name out=w308:refnum<visa-resource-name>, error out=w306:errorcluster)  [unwired: 1 out]
      }
      frame #1 {
      }
    }
    n138 = Divide(x=1000.0, y=w294) -> (x/y=w292:dbl)
    n139 = local read "stop"() -> (w295:bool)
    n140 = Wait (ms)(milliseconds to wait=w292) -> ()  [unwired: 1 out]
  }
  n141 = VISA Close(VISA resource name=w6, error in (no error)=w1) -> ()  [unwired: 1 out]
